vi "DHE_stop_sequence.vi"(0 "fd in":i32, 11 "error in (no error)":errorcluster) -> (4 "fd out":i32, 6 "response":i32, 15 "error out":errorcluster)   [LabVIEW 2016]
doc: "This VI closes the I/O interface with the instrument."
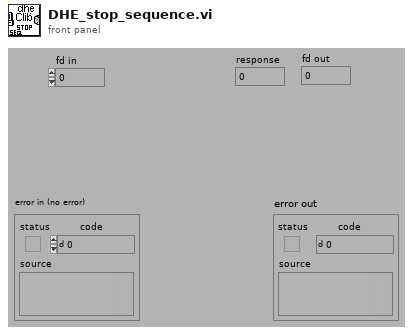
[diagram p1: front panel]
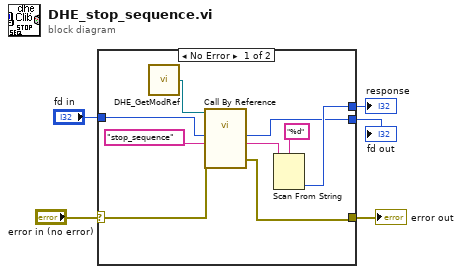
[diagram p0: block diagram]
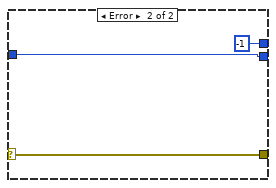
[diagram p2: hidden frame]
diagram:
  n1 = case shown="No Error" "error in (no error)" {
    selector: "error in (no error)" -> [w9 w17]
    tunnel: [w8 w17] -> w5
    tunnel: "fd in" -> [w10 w16]
    tunnel: [w7 -1] -> w2
    tunnel: [w6 w16] -> w1
    frame No Error {
      n2 = call "DHE_GetModRef.vi"() -> ("DHE_ModRef"=w14:refnum<vi>)  [unwired: 9 out]
      n3 = call-by-ref "?"(reference=w14, "error in (no error)"=w9, "function"="stop_sequence", "fd in"=w10) -> ("error out"=w8:errorcluster, "str result"=w12:string, "fd out"=w6:i32)  [unwired: 6 in, 3 out]
      n4 = Scan From String(format string="%d", input string=w12) -> (output 1=w7:i32)  [unwired: 2 in, 4 out]
    }
    frame Error {
    }
  }
  "error out" <- w5
  "response" <- w2
  "fd out" <- w1
